vi "Scanning Volts to Microns.vi"() -> (0 "Scanning Conversions OUT":T1)   [LabVIEW 2014]
uses:
  Scanning Conversions.ctl
panel:
  in  "Scanning Conversions IN":T1
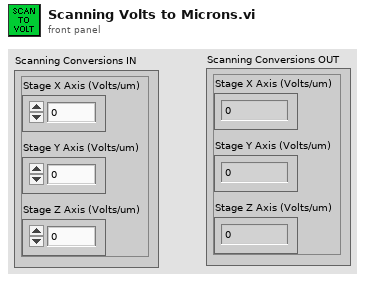
[diagram p1: front panel]
types:
  T1 = typedef "Scanning Conversions.ctl" = cluster{"Stage X Axis (Volts/um)":dbl, "Stage Y Axis (Volts/um)":dbl, "Stage Z Axis (Volts/um)":dbl}
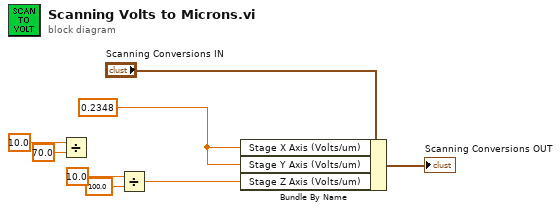
[diagram p0: block diagram]
diagram:
  w1 = 0.2348
  n1 = Divide(x=10.0, y=70.0) -> ()  [unwired: 1 out]
  n2 = Divide(x=10.0, y=100.0) -> (x/y=w3:dbl)
  n3 = Bundle By Name(cluster="Scanning Conversions IN", "Stage X Axis (Volts/um)"=w1, "Stage Y Axis (Volts/um)"=w1, "Stage Z Axis (Volts/um)"=w3) -> (→"Scanning Conversions OUT":T1)
